vi "3.4.vi"() -> ()   [LabVIEW 2017]
panel:
  in  "尾":string
  in  "头":string
  out "字符串长度":i32
  out "连接后的字符串":string
  in  "数值":dbl
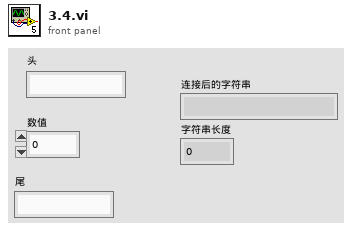
[diagram p1: front panel]
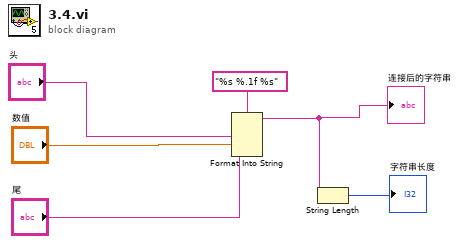
[diagram p0: block diagram]
diagram:
  n1 = Format Into String(format string="%s %.1f %s" ("格式字符串"), "头", "数值", "尾") -> (resulting string=w5:string)  [unwired: 2 in, 1 out]
  "连接后的字符串" <- w5
  n2 = String Length(string=w5) -> (length=→"字符串长度":i32)
